vi "Beacon_Scale_to_Distance_R0.vi"(10 "Scale - In":dbl, 11 "Current Template - In":T1(ring)) -> (3 "Distance - Out":sgl)   [LabVIEW 2015]
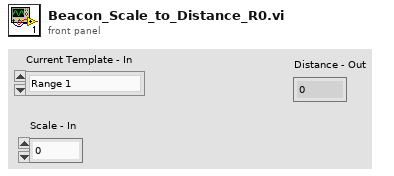
[diagram p1: front panel]
types:
  T1 = enum16{"Range 1", "Range 2", "Range 3", "Range 0"}
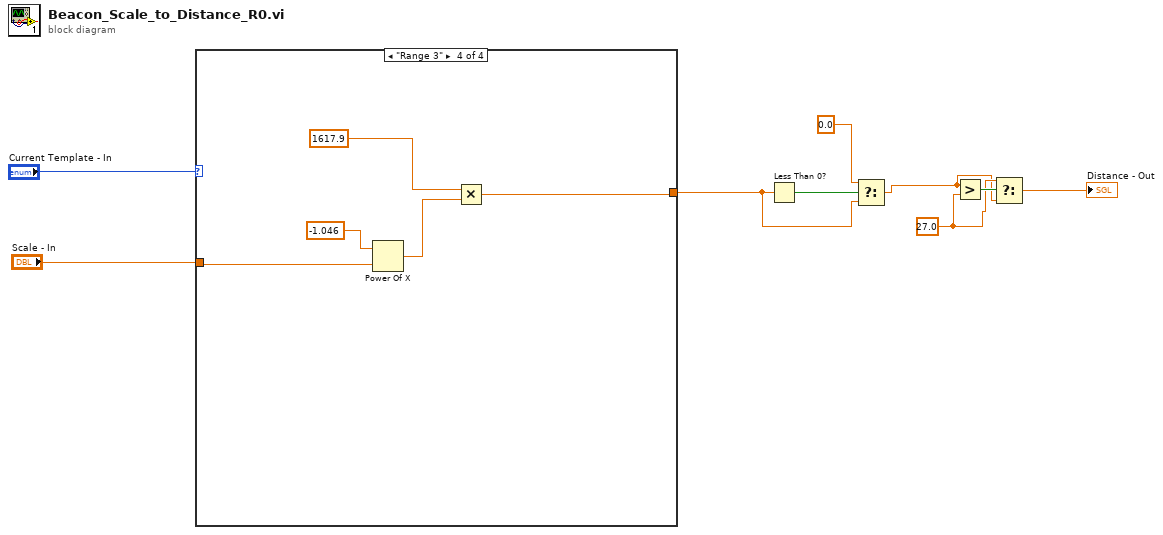
[diagram p0: block diagram]
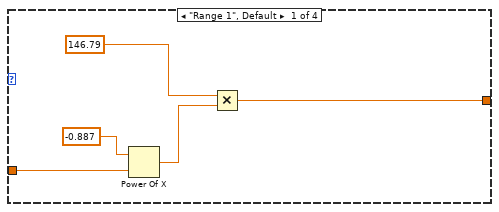
[diagram p2: hidden frame]
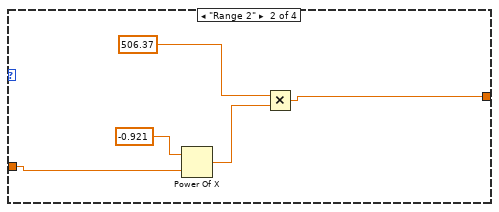
[diagram p3: hidden frame]
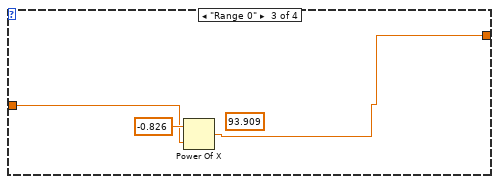
[diagram p4: hidden frame]
diagram:
  w2 = sgl 27.0
  n1 = case shown="\"Range 3\"" "Current Template - In" {
    tunnel: "Scale - In" -> [w13 w16 w21 w24]
    tunnel: [w10 w15 w20 w23] -> w5
    frame "Range 1", Default {
      n2 = Power Of X(1:w13, 2:-0.887) -> (0:w11:dbl)
      n3 = Multiply(x=146.79, y=w11) -> (x*y=w10:dbl)
    }
    frame "Range 2" {
      n4 = Power Of X(1:w16, 2:-0.921) -> (0:w17:dbl)
      n5 = Multiply(x=506.37, y=w17) -> (x*y=w15:dbl)
    }
    frame "Range 0" {
      (unwired) 93.909
      n6 = Power Of X(1:w21, 2:-0.826) -> (0:w20:dbl)
    }
    frame "Range 3" {
      n7 = Power Of X(1:w24, 2:-1.046) -> (0:w25:dbl)
      n8 = Multiply(x=1617.9, y=w25) -> (x*y=w23:dbl)
    }
  }
  n9 = Less Than 0?(x=w5) -> (x < 0?=w6:bool)
  n10 = Select(t=sgl 0.0, s=w6, f=w5) -> (s? t:f=w1:dbl)
  n11 = Greater?(x=w1, y=w2) -> (0:w4:bool)
  n12 = Select(t=w2, s=w4, f=w1) -> (s? t:f=→"Distance - Out":dbl)
